vi "XML.Limits.Generate.FindSeqNameByRoot.vi"(10 "root":string, 11 "seqs in":T1[](array[typedef])) -> (3 "sequence":string)   [LabVIEW 2019, in "Tools.lvlib"]
uses:
  Tools.lvlib
  TestStand/Export limits/controls/TS.Seq.Step.Type.ctl
  TestStand/Export limits/controls/TS.Seq.Type.ctl
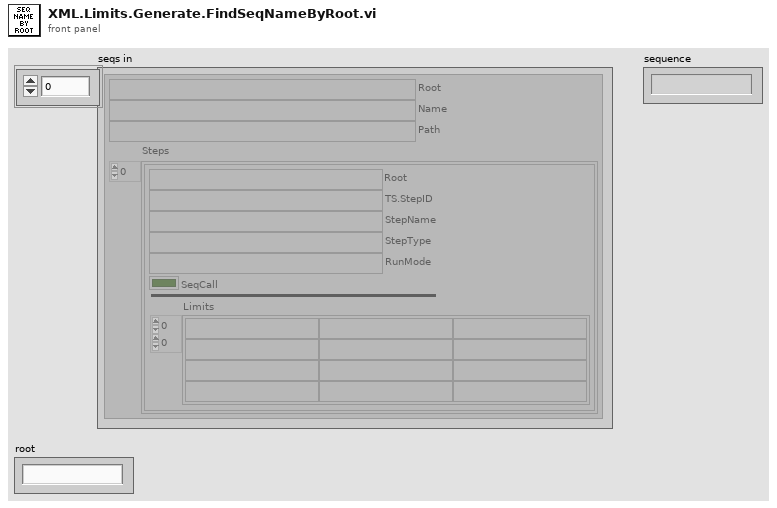
[diagram p1: front panel]
types:
  T1 = typedef "TS.Seq.Type.ctl" = cluster{"Root":string, "Name":string, "Path":string, "Steps":T2[]}
  T2 = typedef "TS.Seq.Step.Type.ctl" = cluster{"Root":string, "TS.StepID":string, "StepName":string, "StepType":string, "RunMode":string, "SeqCall":bool, "Limits":string[][]}
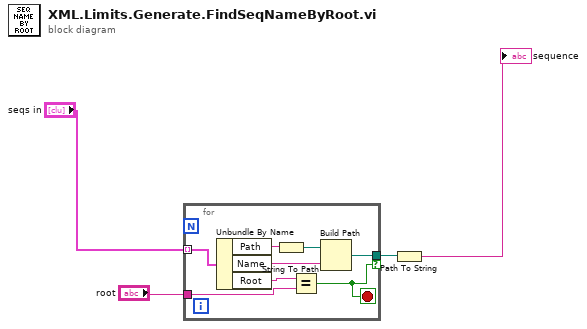
[diagram p0: block diagram]
diagram:
  n1 = for {
    tunnel: "seqs in" -> [w12] mode=indexing
    tunnel: [w8] -> w3 if=w5
    tunnel: "root" -> [w6]
    stop <- w5 stop-if-true
    n2 = Unbundle By Name(w12) -> ("Path"=w11:string, "Name"=w9:string, "Root"=w7:string)
    n3 = String To Path(string=w11) -> (path=w10:path)
    n4 = Equal?(x=w7, y=w6) -> (x = y?=w5:bool)
    n5 = Build Path(base path=w10, name or relative path=w9) -> (appended path=w8:path)
  }
  n6 = Path To String(path=w3) -> (string=→"sequence":string)
